vi "CompareToDigits.vi"(1 "Digits":i32, 2 "A":T1, 3 "A 2":T1) -> (0 "Equal":bool)   [LabVIEW 2025]
uses:
  Number.ctl
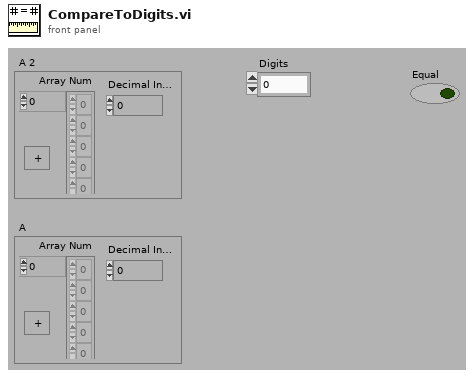
[diagram p1: front panel]
types:
  T1 = typedef "Number.ctl" = cluster{"Array Num":i8[], "Decimal Index":i32, "stop":bool}
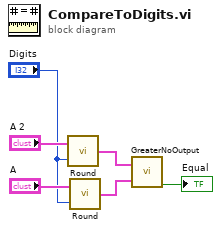
[diagram p0: block diagram]
diagram:
  n1 = call "Round.vi"("Digits"="Digits", "A"="A 2") -> ("A rounded to Digits"=w2:T1)
  n2 = call "Round.vi"("Digits"="Digits", "A"="A") -> ("A rounded to Digits"=w1:T1)
  n3 = call "GreaterNoOutput.vi"("A"=w2, "B"=w1) -> ("Equal"=→"Equal":bool)  [unwired: 1 in, 2 out]
